vi "GOOP_GetClassReaderByClassRef.vi"(1 "LVClassLibrary Refnum":refnum<vi>, 5 "error in (no error)":errorcluster) -> (14 "ClassReaderNative out":refnum<class "ClassReaderNative.lvclass">, 19 "error out":errorcluster)   [LabVIEW 2020]
uses:
  ClassProviders/Provider_LvNativeClass/ClassReaderNative_class/ClassReaderNative.lvclass
  ClassProviders/Provider_LvNativeClass/LvNativeProviderName.ctl
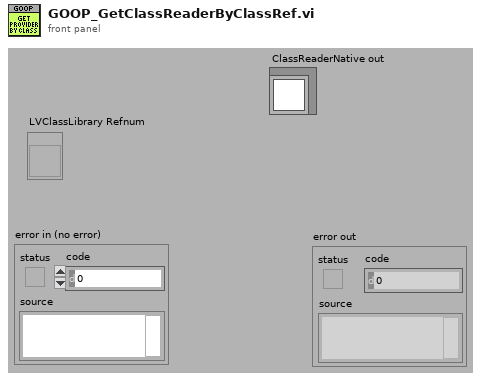
[diagram p1: front panel]
types:
  T1 = typedef "LvNativeProviderName.ctl" = enum16{"Endevo LabVIEW Native"}
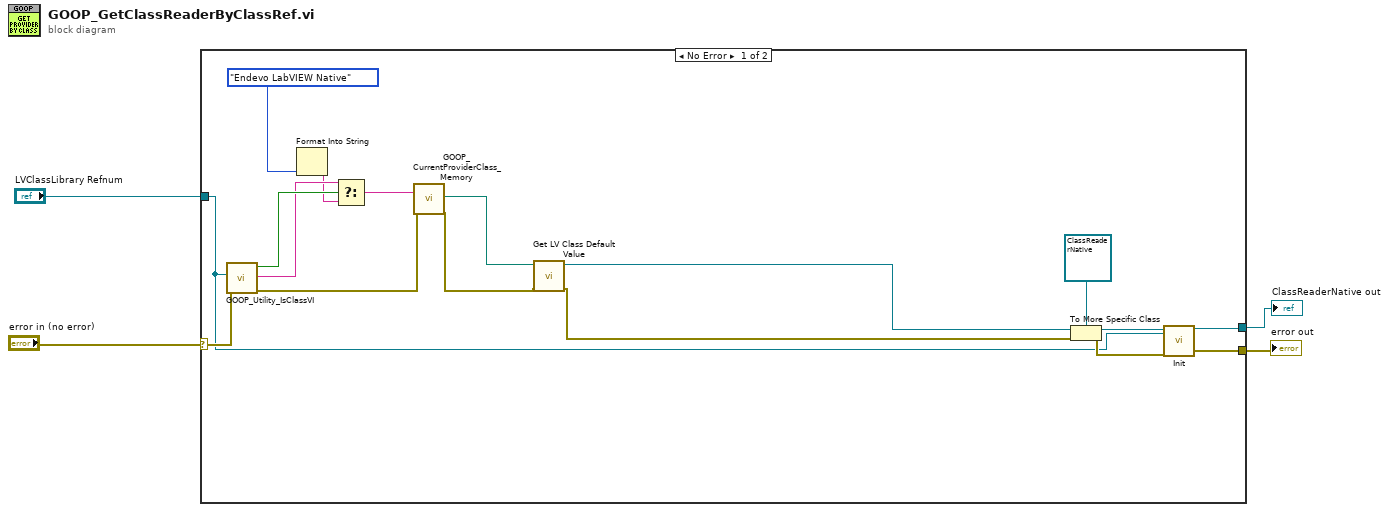
[diagram p0: block diagram]
diagram:
  n1 = case shown="No Error" "error in (no error)" {
    selector: "error in (no error)" -> [w21 w22]
    tunnel: "LVClassLibrary Refnum" -> [w10 _]
    tunnel: [w12 w22] -> w2
    tunnel: [w13 _] -> w1
    frame No Error {
      n2 = call "GOOP_Utility_IsClassVI.vi"("error in (no error)"=w21, "ProjectItem"=w10) -> ("error out"=w20:errorcluster, "ClassProvider"=w18:string, "Is Class VI?"=w19:bool)  [unwired: 4 in, 3 out]
      n3 = Format Into String(LvNativeProviderName."Endevo LabVIEW Native" ("ProviderName")) -> (resulting string=w15:string)  [unwired: 3 in, 1 out]
      n4 = Select(t=w18, s=w19, f=w15) -> (s? t:f=w17:string)
      n5 = call "GOOP_CurrentProviderClass_Memory.vi"("GetThisClassProvidersPaths(Returns the default providor if not wired)"=w17, "error in (no error)"=w20) -> ("ClassProviderClassReaderPath"=w8:path, "error out"=w5:errorcluster)  [unwired: 11 in, 5 out]
      n6 = call <vilib>:"Get LV Class Default Value.vi"("error in (no error)"=w5, "class path"=w8) -> ("error out"=w6:errorcluster, "object"=w7:refnum<class>)  [unwired: 8 in]
      n7 = To More Specific Class(target class=refnum<class "ClassReaderNative.lvclass"> refnum ("ClassReaderNative.lvclass"), reference=w7, error in=w6) -> (specific class reference=w11:refnum<class "ClassReaderNative.lvclass">, error out=w14:errorcluster)
      n8 = call-dynamic "Init.vi"("ClassReaderNative in"=w11, "LvClassRef"=w10, "error in (no error)"=w14) -> ("ClassReaderNative out"=w13:refnum<class "ClassReaderNative.lvclass">, "error out"=w12:errorcluster)  [unwired: 15 in]
    }
    frame Error {
    }
  }
  "error out" <- w2
  "ClassReaderNative out" <- w1
